vi "Drive.vi"(0 "b,a,d,c":cluster{"b":dbl, "a":dbl, "d":dbl, "c":dbl}, 1 "Swerve DevRef":T1={"DeviceStatus"={"status"=FALSE, "code"=0, "source"=""}, "Type"=enum."PWM", "PWM"={"PWM Channel"=enum."PWM 1", "DeadBand"={"Name"="", "maxPositivePwm"=0, "minPositivePwm"=0, "centerPwm"=0, "maxNegativePwm"=0, "minNegativePwm"=0, "angularRange"=0}}, "CAN"={"Device Number"=0, "SetOutput VI Ref"=variant(enum8{"Percent VBus", "Current", "Speed", "Position", "Voltage"} enum."Percent VBus"), "GetOutput VI Ref"=variant(refnum<k1> refnum), "Enable VI Ref"=variant(dbl 12.0), "Disable VI Ref"=variant(enum8{"Percent VBus", "Speed", "Position", "Slave", "Unchanged / Invalid", "Voltage Compensation", "Current", "Motion Profile"} enum."Percent VBus"), "Data"=variant}, "Invert"=FALSE}, 2 "Wheel DevRef":T1={"DeviceStatus"={"status"=FALSE, "code"=0, "source"=""}, "Type"=enum."PWM", "PWM"={"PWM Channel"=enum."Invalid", "DeadBand"={"Name"="", "maxPositivePwm"=0, "minPositivePwm"=0, "centerPwm"=0, "maxNegativePwm"=0, "minNegativePwm"=0, "angularRange"=0}}, "CAN"={"Device Number"=0, "SetOutput VI Ref"=variant(refnum<vi> refnum), "GetOutput VI Ref"=variant(refnum<vi> refnum), "Enable VI Ref"=variant(refnum<vi> refnum), "Disable VI Ref"=variant(refnum<vi> refnum), "Data"=variant}, "Invert"=FALSE}, 3 "error in":errorcluster, 4 "Index":i32) -> (5 "Swerve Speed":dbl, 6 "Wheel Speed":dbl, 7 "error out":errorcluster)   [LabVIEW 2016]
uses:
  <vilib>/Rock Robotics/WPI/MotorControl/WPI_MotorControlDeviceRef.ctl
  <vilib>/Rock Robotics/WPI/MotorControl/WPI_MotorControlType.ctl
  <vilib>/Rock Robotics/SystemInterfaces/DIO/FPGA_DIOPWMChannel.ctl
  <vilib>/Rock Robotics/WPI/PWM/WPI_PWMDeadband.ctl
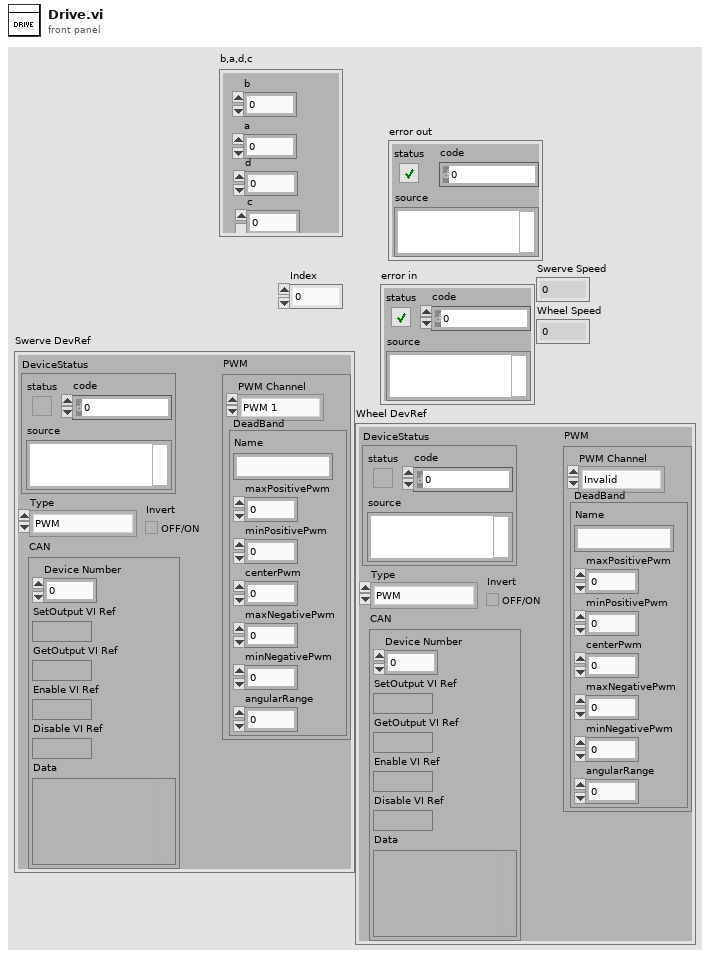
[diagram p1: front panel]
types:
  T1 = typedef "WPI_MotorControlDeviceRef.ctl" = cluster{"DeviceStatus":errorcluster, "Type":T2, "PWM":cluster{"PWM Channel":T3, "DeadBand":T4}, "CAN":cluster{"Device Number":u8, "SetOutput VI Ref":variant, "GetOutput VI Ref":variant, "Enable VI Ref":variant, "Disable VI Ref":variant, "Data":variant}, "Invert":bool}
  T2 = typedef "WPI_MotorControlType.ctl" = enum16{"PWM", "CAN"}
  T3 = typedef "FPGA_DIOPWMChannel.ctl" = enum8{"PWM 0", "PWM 1", "PWM 2", "PWM 3", "PWM 4", "PWM 5", "PWM 6", "PWM 7", "PWM 8", "PWM 9", "PWM MXP 0", "PWM MXP 1", "PWM MXP 2", "PWM MXP 3", "PWM MXP 4", "PWM MXP 5", "PWM MXP 6", "PWM MXP 7", "PWM MXP 8", "PWM MXP 9", "Invalid"}
  T4 = typedef "WPI_PWMDeadband.ctl" = cluster{"Name":string, "maxPositivePwm":i32, "minPositivePwm":i32, "centerPwm":i32, "maxNegativePwm":i32, "minNegativePwm":i32, "angularRange":u16}
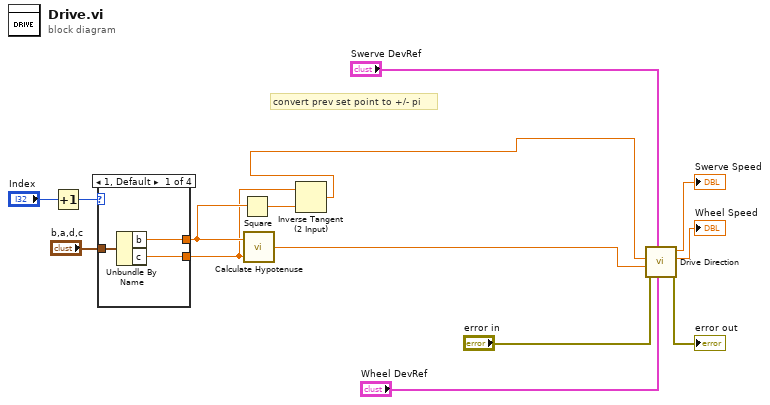
[diagram p0: block diagram]
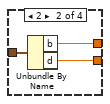
[diagram p2: hidden frame]
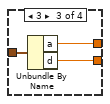
[diagram p3: hidden frame]
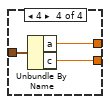
[diagram p4: hidden frame]
diagram:
  # "convert prev set point to +/- pi"
  n1 = Increment(x="Index") -> (x+1=w3:i32)
  n2 = case shown="1, Default" w3 {
    tunnel: "b,a,d,c" -> [w17 w20 w23 w26]
    tunnel: [w16 w19 w22 w25] -> w11
    tunnel: [w15 w18 w21 w24] -> w10
    frame 1, Default {
      n3 = Unbundle By Name(w17) -> ("b"=w16:dbl, "c"=w15:dbl)
    }
    frame 2 {
      n4 = Unbundle By Name(w20) -> ("b"=w19:dbl, "d"=w18:dbl)
    }
    frame 3 {
      n5 = Unbundle By Name(w23) -> ("a"=w22:dbl, "d"=w21:dbl)
    }
    frame 4 {
      n6 = Unbundle By Name(w26) -> ("a"=w25:dbl, "c"=w24:dbl)
    }
  }
  n7 = Square(x=w11) -> (x^2=w12:dbl)
  n8 = call "Calculate Hypotenuse.vi"("Y"=w10, "X"=w11) -> ("Hypotenuse"=w2:dbl)
  n9 = Inverse Tangent (2 Input)(1:w12, 2:w10) -> (0:w1:dbl)
  n10 = call "Drive Direction.vi"("Wheel DevRef"="Wheel DevRef", "Swerve DevRef"="Swerve DevRef", "error in"="error in", "Wheel Power"=w2, "Desired direction (radians)"=w1) -> ("error out"=→"error out":errorcluster, "Wheel Speed"=→"Wheel Speed":dbl, "Swerve Speed"=→"Swerve Speed":dbl)  [unwired: 4 in]
